vi "Controller Orbit Correction Matrix Calculation.vi"(5 "Corrector Planes":enum8{"H", "V"}[](array[ring]), 6 "Decouple H-V? (true)":bool=TRUE, 7 "BPM Reading Planes":enum8{"H", "V"}[](array[ring]), 8 "error in (no error)":errorcluster, 9 "Selected Correctors":u32[](array[numeric]), 10 "Selected BPM Readings":u32[](array[numeric]), 11 "Response Matrix":dbl[][](array[numeric])) -> (0 "error out":errorcluster, 3 "Correction Matrix":dbl[][](array[numeric]))   [LabVIEW 2011, in "Controller VIs.lvlib"]
doc: "Calculates the Correction Matrix for a given Response Matrix. The Singular Value Decomposition (SVD) method is used as inversion algorithm. The Correction Matrix has as many rows as indicated by the Selected Correctors and as many columns as indicated by the Selected BPMs. By default, the Correction Matrix has decoupled response for the Horizontal and Vertical planes."
uses:
  Controller VIs.lvlib
  <vilib>/Analysis/_algsub.llb/Real PseudoInverse Matrix.vi
  <vilib>/Analysis/NI_AALPro.lvlib
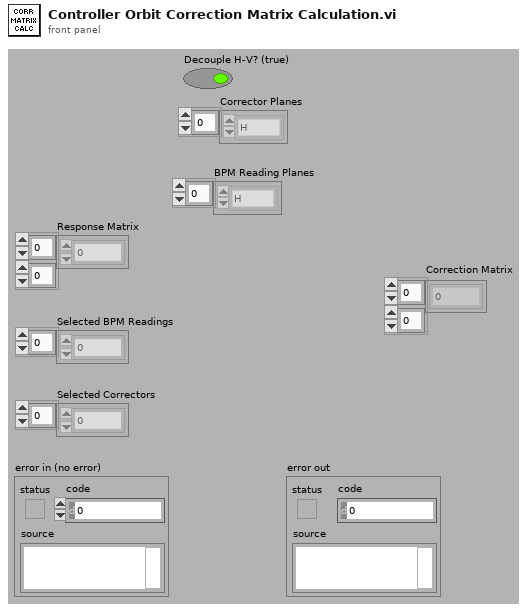
[diagram p1: front panel]
types:
  T1 = typedef "NI_Matrix.lvlib/RealMatrix.ctl" = dbl[][]
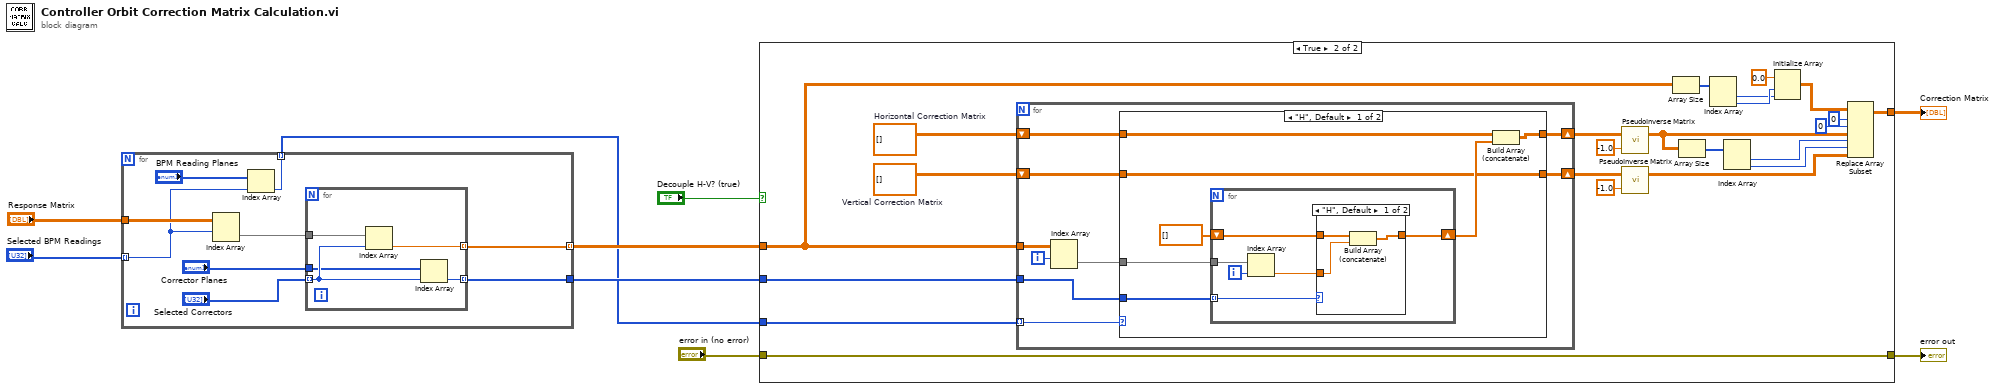
[diagram p0: block diagram]
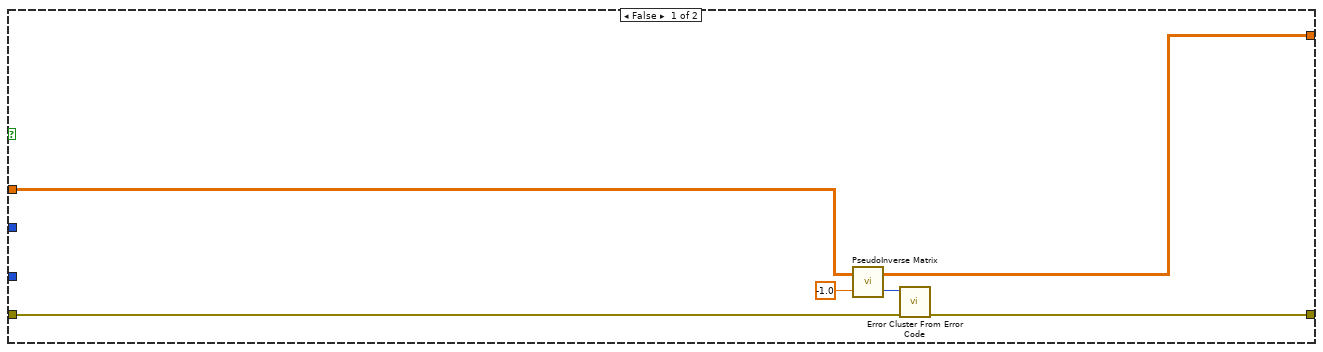
[diagram p2: hidden frame]
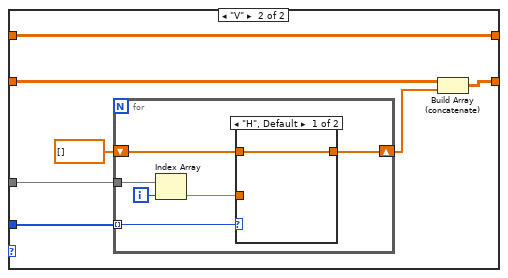
[diagram p4: hidden frame]
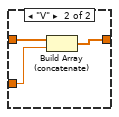
[diagram p5: hidden frame]
diagram:
  n1 = for {
    tunnel: "Response Matrix" -> [w18]
    tunnel: "Selected BPM Readings" -> [w14] mode=indexing
    tunnel: [w16] -> w8 mode=indexing
    tunnel: [w15] -> w6
    tunnel: [w13] -> w5 mode=indexing
    n2 = Index Array(array=w18, index (row)=w14) -> (element=w17:dbl[])  [unwired: 1 in]
    n3 = Index Array(array="BPM Reading Planes", index=w14) -> (element=w13:enum8{"H", "V"})
    n4 = for {
      tunnel: w17 -> [w23]
      tunnel: "Selected Correctors" -> [w21] mode=indexing
      tunnel: [w22] -> w16 mode=indexing
      tunnel: [w20] -> w15 mode=indexing
      tunnel: "Corrector Planes" -> [w19]
      n5 = Index Array(array=w23, index=w21) -> (element=w22:dbl)
      n6 = Index Array(array=w19, index=w21) -> (element=w20:enum8{"H", "V"})
    }
  }
  n7 = case shown="True" "Decouple H-V? (true)" {
    tunnel: w8 -> [w24 w42]
    tunnel: w6 -> [_ w41]
    tunnel: w5 -> [_ w40]
    tunnel: "error in (no error)" -> [w27 w30]
    tunnel: [w26 w30] -> w3
    tunnel: [w25 w33] -> w2
    frame False {
      n8 = call-poly <vilib>:"PseudoInverse Matrix.vi"("tolerance"=-1.0, "Input Matrix"=w24) -> ("error"=w28:i32, "PseudoInverse Matrix"=w25:T1)
      n9 = call <vilib>:"Error Cluster From Error Code.vi"("error in (no error)"=w27, "error code (0)"=w28) -> ("error out"=w26:errorcluster)  [unwired: 7 in]
    }
    frame True {
      w51 = dbl[][] []  # Vertical Correction Matrix
      w52 = dbl[][] []  # Horizontal Correction Matrix
      n10 = for {
        tunnel: w40 -> [w58] mode=indexing
        tunnel: w42 -> [w61]
        shift-right: [w56] -> w39
        shift-left: w52 -> [w57]
        shift-right: [w55] -> w36
        shift-left: w51 -> [w54]
        tunnel: w41 -> [w53]
        i -> [w60]
        n11 = Index Array(array=w61, index (row)=w60) -> (element=w59:dbl[])  [unwired: 1 in]
        n12 = case shown="\"H\", Default" w58 {
          tunnel: w59 -> [w68 w82]
          tunnel: w57 -> [w65 w85]
          tunnel: [w64 w85] -> w56
          tunnel: w54 -> [w62 w80]
          tunnel: [w62 w81] -> w55
          tunnel: w53 -> [w63 w83]
          frame "H", Default {
            n13 = for {
              tunnel: w63 -> [w72] mode=indexing
              tunnel: w68 -> [w73]
              shift-right: [w70] -> w66
              shift-left: dbl[] [] -> [w69]
              i -> [w74]
              n14 = Index Array(array=w73, index=w74) -> (element=w71:dbl)
              n15 = case shown="\"H\", Default" w72 {
                tunnel: w71 -> [w77 _]
                tunnel: [w76 w78] -> w70
                tunnel: w69 -> [w75 w78]
                frame "H", Default {
                  n16 = Build Array (concatenate)(w75, w77) -> (w76:dbl[])
                }
                frame "V" {
                }
              }
            }
            n17 = Build Array (concatenate)(w65, w66) -> (w64:dbl[][])
          }
          frame "V" {
            n18 = for {
              tunnel: w83 -> [w89] mode=indexing
              tunnel: w82 -> [w90]
              shift-right: [w87] -> w79
              shift-left: dbl[] [] -> [w86]
              i -> [w91]
              n19 = Index Array(array=w90, index=w91) -> (element=w88:dbl)
              n20 = case shown="\"H\", Default" w89 {
                tunnel: w88 -> [_ w95]
                tunnel: [w92 w94] -> w87
                tunnel: w86 -> [w92 w93]
                frame "H", Default {
                }
                frame "V" {
                  n21 = Build Array (concatenate)(w93, w95) -> (w94:dbl[])
                }
              }
            }
            n22 = Build Array (concatenate)(w80, w79) -> (w81:dbl[][])
          }
        }
      }
      n23 = call-poly <vilib>:"PseudoInverse Matrix.vi"("tolerance"=-1.0, "Input Matrix"=w39) -> ("PseudoInverse Matrix"=w32:T1)  [unwired: 1 out]
      n24 = call-poly <vilib>:"PseudoInverse Matrix.vi"("tolerance"=-1.0, "Input Matrix"=w36) -> ("PseudoInverse Matrix"=w31:T1)  [unwired: 1 out]
      n25 = Array Size(array=w42) -> (size(s)=w43:i32[])
      n26 = Array Size(array=w32) -> (size(s)=w48:i32[])
      n27 = Index Array(array=w43) -> (element #1=w34:i32, element #2=w35:i32)  [unwired: 2 in]
      n28 = Index Array(array=w48) -> (element #1=w49:i32, element #2=w50:i32)  [unwired: 2 in]
      n29 = Initialize Array(0.0 ("element"), w35, w34) -> (w45:dbl[][])
      n30 = Replace Array Subset(array=w45, new element #1=w32, index (row) #1=0 ("row 1"), index (col) #1=0 ("column 1"), new element #2=w31, index (row) #2=w49, index (col) #2=w50) -> (w33:T1)
    }
  }
  "Correction Matrix" <- w2
  "error out" <- w3
